vi "TesteLeds.vi"() -> ()   [LabVIEW 2018]
panel:
  out "ledP0":bool
  out "ledP1":bool
  out "ledP2":bool
  out "ledP3":bool
  out "ledP4":bool
  out "ledP5":bool
  out "ledP6":bool
  out "ledP7":bool
  out "ledP8":bool
  out "ledP10":bool
  out "ledP11":bool
  out "ledP12":bool
  out "ledP13":bool
  out "ledP14":bool
  out "ledP15":bool
  out "ledP9":bool
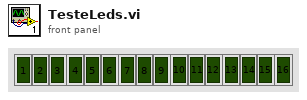
[diagram p1: front panel]
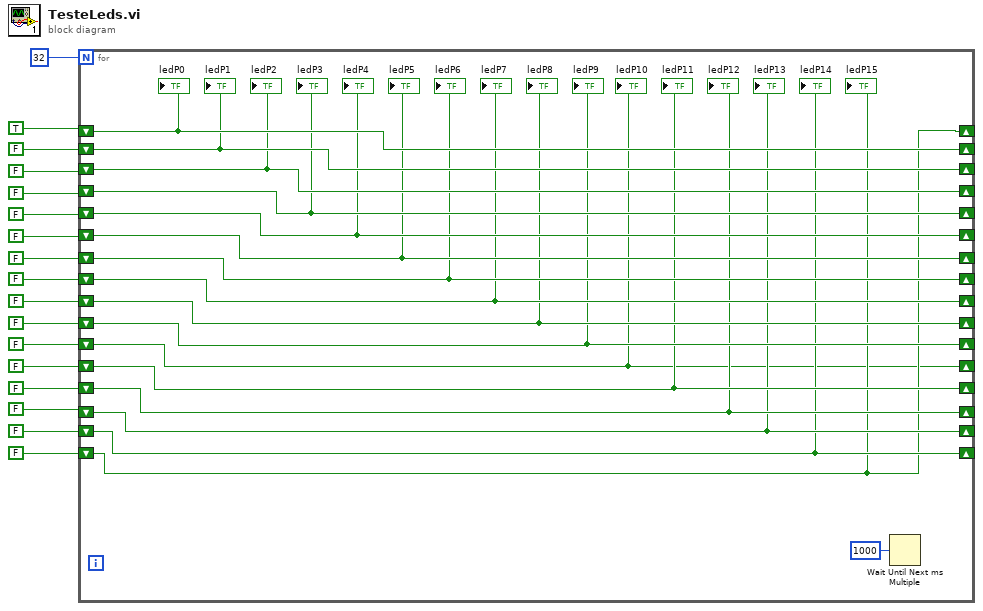
[diagram p0: block diagram]
diagram:
  n1 = for {
    N: 32 -> [_]
    shift-right: [w19] -> _
    shift-left: TRUE -> [w33]
    shift-right: [w33] -> _
    shift-left: FALSE -> [w32]
    shift-right: [w32] -> _
    shift-left: FALSE -> [w31]
    shift-right: [w31] -> _
    shift-left: FALSE -> [w30]
    shift-right: [w30] -> _
    shift-left: FALSE -> [w29]
    shift-right: [w29] -> _
    shift-left: FALSE -> [w28]
    shift-right: [w28] -> _
    shift-left: FALSE -> [w27]
    shift-right: [w27] -> _
    shift-left: FALSE -> [w26]
    shift-right: [w26] -> _
    shift-left: FALSE -> [w25]
    shift-right: [w25] -> _
    shift-left: FALSE -> [w24]
    shift-right: [w24] -> _
    shift-left: FALSE -> [w18]
    shift-right: [w18] -> _
    shift-left: FALSE -> [w23]
    shift-right: [w23] -> _
    shift-left: FALSE -> [w22]
    shift-right: [w22] -> _
    shift-left: FALSE -> [w21]
    shift-right: [w21] -> _
    shift-left: FALSE -> [w20]
    shift-right: [w20] -> _
    shift-left: FALSE -> [w19]
    n2 = Wait Until Next ms Multiple(millisecond multiple=u32 1000) -> ()  [unwired: 1 out]
    "ledP0" <- w33
    "ledP1" <- w32
    "ledP2" <- w31
    "ledP3" <- w30
    "ledP4" <- w29
    "ledP5" <- w28
    "ledP6" <- w27
    "ledP7" <- w26
    "ledP8" <- w25
    "ledP9" <- w24
    "ledP10" <- w18
    "ledP11" <- w23
    "ledP12" <- w22
    "ledP13" <- w21
    "ledP14" <- w20
    "ledP15" <- w19
  }
